vi "Status Read Connects.vi"(8 "error in (no error)":errorcluster, 9 "Lenght (1)":i32=1, 10 "N (0)":i32, 11 "Status References":T1[](array[typedef])) -> (0 "error out":errorcluster, 1 "Connect":bool[](array[boolean]))   [LabVIEW 2019, in "Status.lvlib"]
uses:
  Status.lvlib
  Ctl/control.ctl
  Ctl/State.ctl
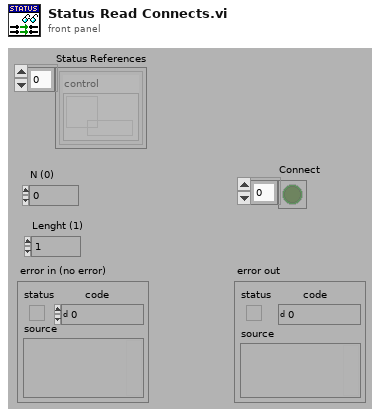
[diagram p1: front panel]
types:
  T1 = typedef "Status.lvlib/control.ctl" = cluster{"control":refnum<data-value>}
  T2 = typedef "Status.lvlib/State.ctl" = enum8{"initialization", "redefine", "standby", "connect", "wait to reconnect", "wait to reset timeout", "configure", "requests", "close connection", "stop"}
  T3 = cluster{"set_state":cluster{"Start":bool, "WrEn":bool, "Stop":bool}, "state":cluster{"errors":i32, "connect":bool, "state":T2}}
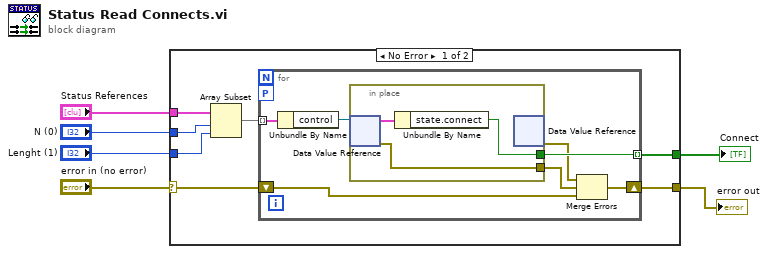
[diagram p0: block diagram]
diagram:
  n1 = case shown="No Error" "error in (no error)" {
    selector: "error in (no error)" -> [w8 w24]
    tunnel: [w7 w24] -> w6
    tunnel: [w13 _] -> w3
    tunnel: "N (0)" -> [w11 _]
    tunnel: "Status References" -> [w12 _]
    tunnel: "Lenght (1)" -> [w10 _]
    frame No Error {
      n2 = Array Subset(array=w12, index=w11, length=w10) -> (w9:T1[])
      n3 = for {
        tunnel: [w20] -> w13 mode=indexing
        tunnel: w9 -> [w19] mode=indexing
        shift-right: [w14] -> w7
        shift-left: w8 -> [w15]
        workers-P: _ -> [_]
        n4 = Unbundle By Name(w19) -> ("control"=w18:refnum<data-value>)
        n5 = in-place {
          in-place-border: [w21] -> w20
          in-place-border: [w23] -> w16
          n6 = in-place-dvr #1(w18) -> (w22:T3, w23:errorcluster)
          n7 = Unbundle By Name(w22) -> ("state.connect"=w21:bool)
          n8 = in-place-dvr #1() -> (w17:errorcluster)  [unwired: 1 in, 1 out]
        }
        n9 = Merge Errors(w17, w16, w15) -> (w14:errorcluster)
      }
    }
    frame Error {
    }
  }
  "error out" <- w6
  "Connect" <- w3
